vi "RF机柜开关切换.vi"(6 "COM":u16, 7 "A":u16, 8 "error in":errorcluster caption="error constant", 9 "8x4":refnum<k5>, 10 "RF-B":refnum<k5>, 11 "RF-A":refnum<k5>) -> (0 "error out":errorcluster caption="error constant", 2 "ask":string)   [LabVIEW 2015]
uses:
  server/Global/SeverGlobal.vi
panel:
  out "Isfailed":bool
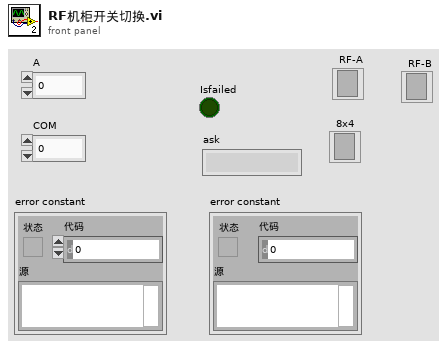
[diagram p1: front panel]
types:
  T1 = enum16{"Standard", "Buffered", "CRLF", "Immediate"}
  T2 = cluster{"IP_A":string, "PORT_A":i32, "IP_B":string, "PORT_B":i32, "IP_CLK":string, "PORT_CLK":i32, "IP_SWITCH":string, "PORT_SWITCH":i32}
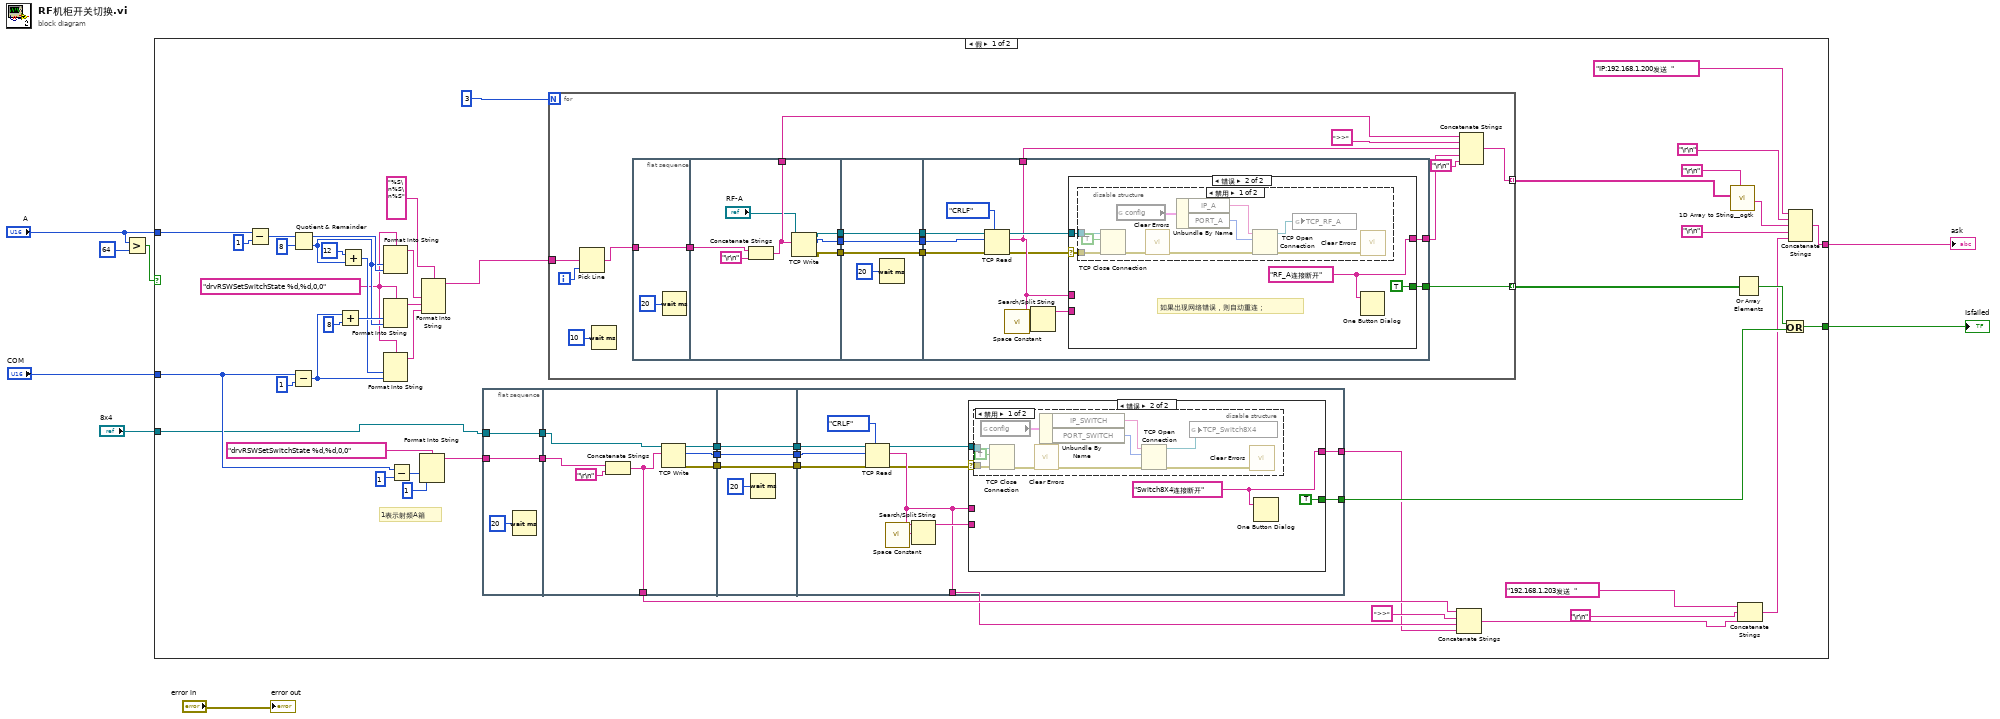
[diagram p0: block diagram]
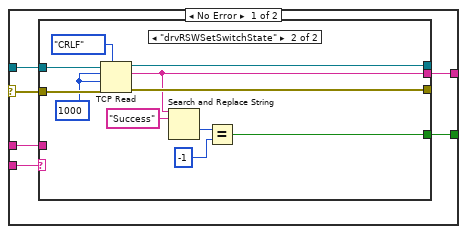
[diagram p2: hidden frame]
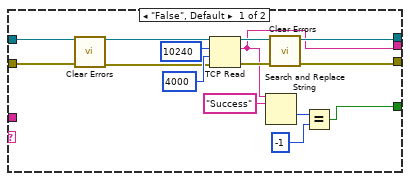
[diagram p3: hidden frame]
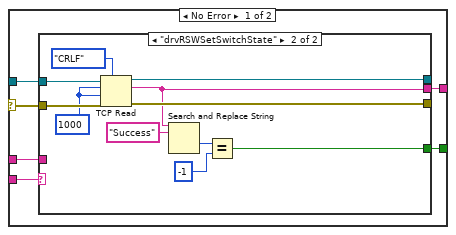
[diagram p5: hidden frame]
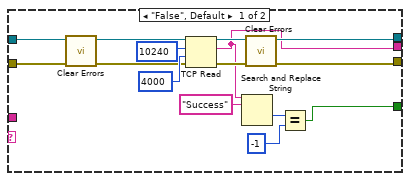
[diagram p6: hidden frame]
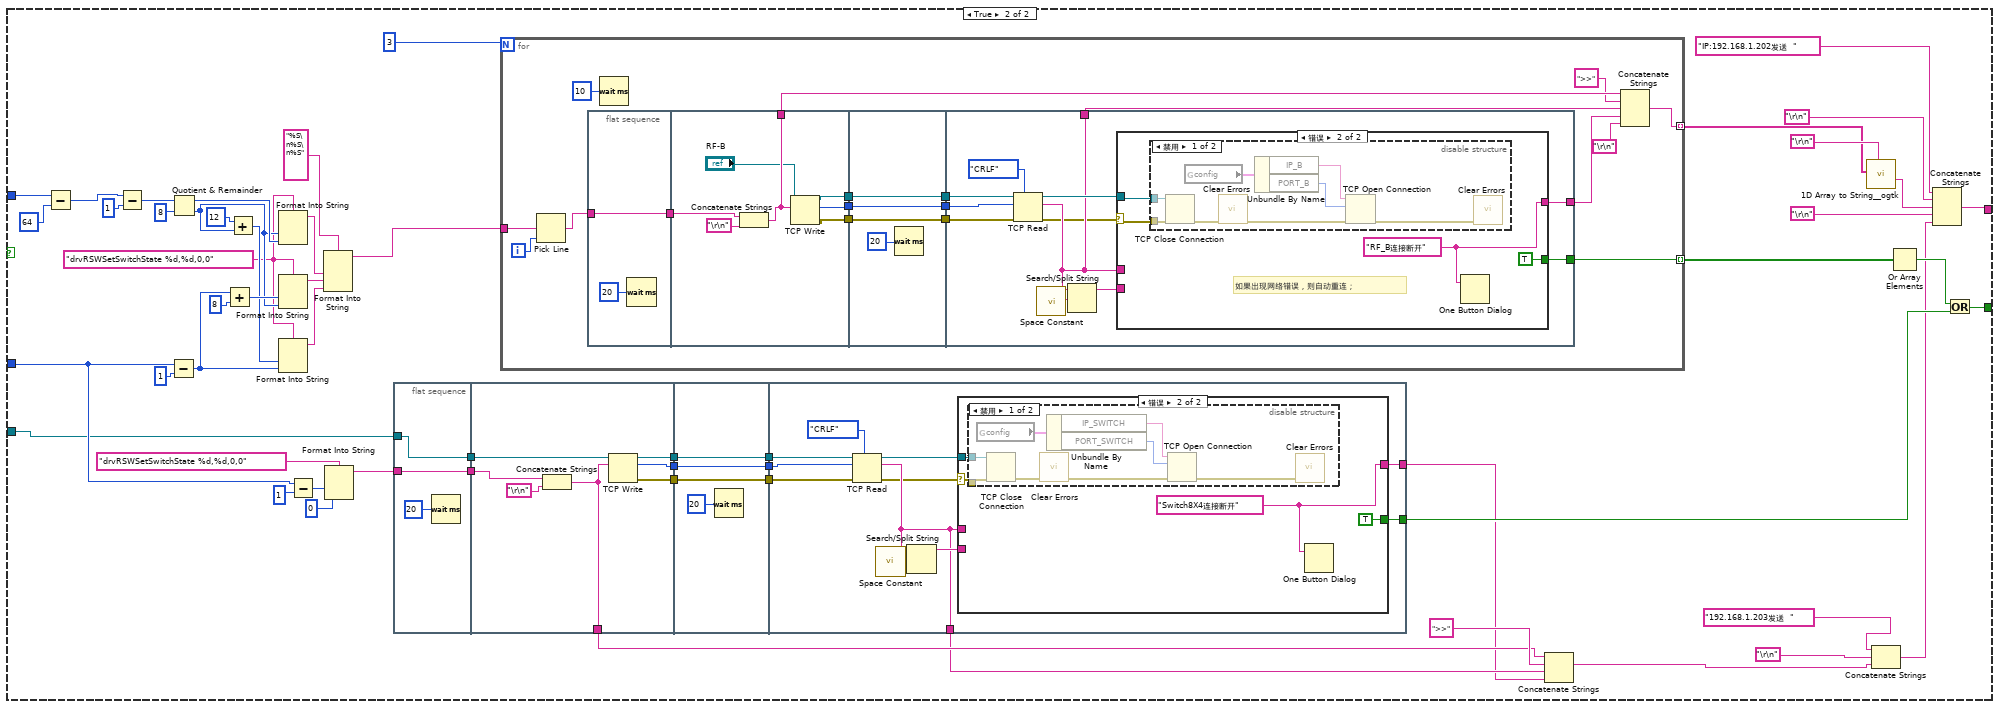
[diagram p8: hidden frame]
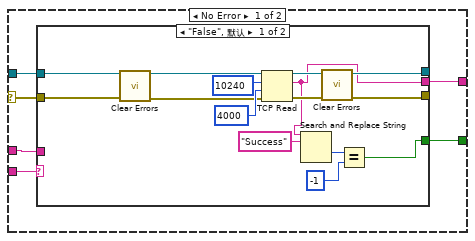
[diagram p9: hidden frame]
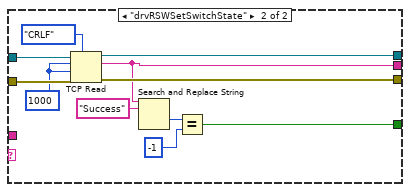
[diagram p10: hidden frame]
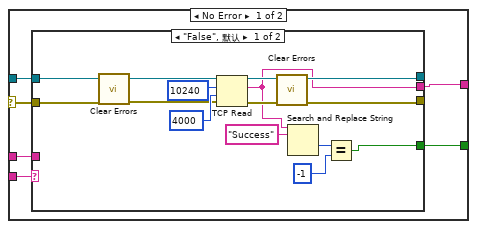
[diagram p12: hidden frame]
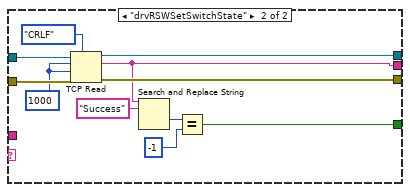
[diagram p13: hidden frame]
diagram:
  n1 = Greater?(x="A", y=u16 64) -> (0:w2:bool)
  n2 = case shown="假" w2 {
    tunnel: "A" -> [w43 w253]
    tunnel: "COM" -> [w39 w239]
    tunnel: [w27 w236] -> w5
    tunnel: [w24 w225] -> w4
    tunnel: "8x4" -> [w10 w218]
    frame False {
      w46 = "drvRSWSetSwitchState %d,%d,0,0" ("格式字符串")
      # "1表示射频A箱"
      n3 = Subtract(x=w43, y=1) -> (x-y=w60:i32)
      n4 = Subtract(x=w39, y=1) -> (x-y=w51:i32)
      n5 = Quotient & Remainder(x=w60, y=8) -> (x-y*floor(x/y)=w55:i32, floor(x/y)=w53:i32)
      n6 = Add(x=w51, y=8) -> (x+y=w54:i32)
      n7 = Add(x=12, y=w53) -> (x+y=w52:i32)
      n8 = Format Into String(format string=w46, w53, w55) -> (resulting string=w49:string)  [unwired: 2 in, 1 out]
      n9 = Format Into String(format string=w46, w54, w53) -> (resulting string=w48:string)  [unwired: 2 in, 1 out]
      n10 = Format Into String(format string=w46, w52, w51) -> (resulting string=w47:string)  [unwired: 2 in, 1 out]
      n11 = Subtract(x=w39, y=1) -> (x-y=w42:i32)
      n12 = Format Into String(format string="drvRSWSetSwitchState %d,%d,0,0" ("格式字符串"), w42, i16 1 ("input 2")) -> (resulting string=w37:string)  [unwired: 2 in, 1 out]
      n13 = Format Into String(format string="%S\n%S\n%S", w49, w48, w47) -> (resulting string=w45:string)  [unwired: 2 in, 1 out]
      n14 = flat-sequence {
        tunnel: w37 -> [w64]
        tunnel: [w64] -> w21
        tunnel: w10 -> [w62]
        tunnel: [w62] -> w9
        tunnel: [w69] -> w36
        tunnel: [w68] -> w35
        tunnel: [w67] -> w31
        tunnel: [w66] -> w14
        tunnel: w21 -> [w71]
        tunnel: w9 -> [w65]
        tunnel: w36 -> [w74]
        tunnel: w35 -> [w73]
        tunnel: [w74] -> w34
        tunnel: [w73] -> w33
        tunnel: [w72] -> w32
        tunnel: w31 -> [w72]
        tunnel: w34 -> [w82]
        tunnel: w33 -> [w81]
        tunnel: w32 -> [w80]
        tunnel: [w79] -> w28
        tunnel: [w78] -> w12
        tunnel: [w77] -> w13
        frame #0 {
          n15 = Wait (ms)(milliseconds to wait=u32 20 ("delay")) -> ()  [unwired: 1 out]
        }
        frame #1 {
          n16 = Concatenate Strings(w71, "\r\n") -> (w66:string)
          n17 = TCP Write(connection ID=w65, data in=w66) -> (connection ID out=w69:refnum<k5>, bytes written=w67:i32, error out=w68:errorcluster)  [unwired: 2 in]
        }
        frame #2 {
          n18 = Wait (ms)(milliseconds to wait=u32 20 ("delay")) -> ()  [unwired: 1 out]
        }
        frame #3 {
          n19 = TCP Read(connection ID=w82, bytes to read=w80, error in (no error)=w81, 7:T1."CRLF" ("mode (standard)")) -> (connection ID out=w86:refnum<k5>, data out=w77:string, error out=w76:errorcluster)  [unwired: 1 in]
          n20 = call <vilib>:"Space Constant.vi"() -> ("String"=w83:string)
          n21 = Search/Split String(string=w77, search string/char (-)=w83) -> (substring before match=w85:string)  [unwired: 1 in, 2 out]
          n22 = case shown="错误" w76 {
            selector: w76 -> [w87 w120]
            tunnel: w86 -> [w92 w119]
            tunnel: w85 -> [w91 _]
            tunnel: [w90 TRUE] -> w79
            tunnel: [w89 w117] -> w78
            tunnel: w77 -> [w88 _]
            frame No Error {
              n23 = case shown="\"drvRSWSetSwitchState\"" w91 {
                tunnel: [w101 w115] -> _
                tunnel: [w100 w114] -> _
                tunnel: w92 -> [w102 w113]
                tunnel: w87 -> [w99 w112]
                tunnel: w88 -> [_ _]
                tunnel: [w93 w107] -> w90
                tunnel: [w94 w106] -> w89
                frame "False", Default {
                  n24 = call <vilib>:"Clear Errors.vi"("error in (no error)"=w99) -> ("error out"=w98:errorcluster)  [unwired: 5 in, 1 out]
                  n25 = TCP Read(connection ID=w102, bytes to read=10240, error in (no error)=w98, 9:4000 ("timeout ms (25000)")) -> (connection ID out=w101:refnum<k5>, data out=w94:string, error out=w104:errorcluster)  [unwired: 1 in]
                  n26 = Search and Replace String(input string=w94, search string="Success") -> (offset past replacement=w95:i32)  [unwired: 6 in, 3 out]
                  n27 = call <vilib>:"Clear Errors.vi"("error in (no error)"=w104) -> ("error out"=w100:errorcluster)  [unwired: 5 in, 1 out]
                  n28 = Equal?(x=w95, y=-1) -> (x = y?=w93:bool)
                }
                frame "drvRSWSetSwitchState" {
                  w111 = 1000 ("timeout ms (25000)")
                  n29 = TCP Read(connection ID=w113, bytes to read=w111, error in (no error)=w112, 7:T1."CRLF" ("mode (standard)"), 9:w111) -> (connection ID out=w115:refnum<k5>, data out=w106:string, error out=w114:errorcluster)
                  n30 = Search and Replace String(input string=w106, search string="Success") -> (offset past replacement=w109:i32)  [unwired: 6 in, 3 out]
                  n31 = Equal?(x=w109, y=-1) -> (x = y?=w107:bool)
                }
              }
            }
            frame Error {
              w117 = "Switch8X4连接断开" ("字符串")
              n32 = disable-structure shown="禁用" {
                disable-tunnel: w120 -> [w123 _]
                disable-tunnel: w119 -> [w122 _]
                frame Disabled {
                  n33 = global read "SeverGlobal.vi" "config"() -> (w126:T2)
                  n34 = TCP Close Connection(connection ID=w122, abort (F)=TRUE ("中止(F)"), error in (no error)=w123) -> (error out=w124:errorcluster)  [unwired: 1 out]
                  n35 = call <vilib>:"Clear Errors.vi"("error in (no error)"=w124) -> ("error out"=w125:errorcluster)  [unwired: 5 in, 1 out]
                  n36 = Unbundle By Name(w126) -> ("IP_SWITCH"=w127:string, "PORT_SWITCH"=w128:i32)
                  n37 = TCP Open Connection(address=w127, remote port or service name=w128, error in (no error)=w125) -> (connection ID=w129:refnum<k5>, error out=w130:errorcluster)  [unwired: 2 in]
                  n38 = global write "SeverGlobal.vi" "TCP_Switch8X4"(w129) -> ()
                  n39 = call <vilib>:"Clear Errors.vi"("error in (no error)"=w130) -> ()  [unwired: 5 in, 2 out]
                }
                frame Enabled {
                }
              }
              n40 = One Button Dialog(message=w117) -> ()  [unwired: 1 in, 1 out]
            }
          }
        }
      }
      n41 = for {
        N: 3 -> [_]
        tunnel: w45 -> [w148]
        tunnel: [w138] -> w30 mode=indexing
        tunnel: [w135] -> w25 mode=indexing
        i -> [w147]
        n42 = Pick Line(multi-line string=w148, line index=w147) -> (output string=w146:string)  [unwired: 1 in]
        n43 = Wait (ms)(milliseconds to wait=u32 10 ("delay")) -> ()  [unwired: 1 out]
        n44 = flat-sequence {
          tunnel: w146 -> [w150]
          tunnel: [w150] -> w134
          tunnel: [w155] -> w144
          tunnel: [w154] -> w142
          tunnel: [w153] -> w140
          tunnel: [w152] -> w132
          tunnel: w134 -> [w156]
          tunnel: [w160] -> w145
          tunnel: w144 -> [w160]
          tunnel: [w159] -> w143
          tunnel: w142 -> [w159]
          tunnel: [w158] -> w141
          tunnel: w140 -> [w158]
          tunnel: w145 -> [w170]
          tunnel: w143 -> [w169]
          tunnel: w141 -> [w168]
          tunnel: [w165] -> w138
          tunnel: [w164] -> w137
          tunnel: [w163] -> w136
          frame #0 {
            n45 = Wait (ms)(milliseconds to wait=u32 20 ("delay")) -> ()  [unwired: 1 out]
          }
          frame #1 {
            n46 = Concatenate Strings(w156, "\r\n") -> (w152:string)
            n47 = TCP Write(connection ID="RF-A", data in=w152) -> (connection ID out=w155:refnum<k5>, bytes written=w154:i32, error out=w153:errorcluster)  [unwired: 2 in]
          }
          frame #2 {
            n48 = Wait (ms)(milliseconds to wait=u32 20 ("delay")) -> ()  [unwired: 1 out]
          }
          frame #3 {
            n49 = TCP Read(connection ID=w170, bytes to read=w169, error in (no error)=w168, 7:T1."CRLF" ("mode (standard)")) -> (connection ID out=w166:refnum<k5>, data out=w164:string, error out=w162:errorcluster)  [unwired: 1 in]
            n50 = call <vilib>:"Space Constant.vi"() -> ("String"=w172:string)
            n51 = Search/Split String(string=w164, search string/char (-)=w172) -> (substring before match=w167:string)  [unwired: 1 in, 2 out]
            n52 = case shown="错误" w162 {
              selector: w162 -> [w173 w205]
              tunnel: w167 -> [w178 _]
              tunnel: w166 -> [w177 w206]
              tunnel: [w176 TRUE] -> w165
              tunnel: w164 -> [w175 _]
              tunnel: [w174 w203] -> w163
              frame No Error {
                n53 = case shown="\"drvRSWSetSwitchState\"" w178 {
                  tunnel: [w187 w201] -> _
                  tunnel: [w186 w200] -> _
                  tunnel: w177 -> [w188 w199]
                  tunnel: w173 -> [w185 w198]
                  tunnel: w175 -> [_ _]
                  tunnel: [w179 w193] -> w176
                  tunnel: [w180 w192] -> w174
                  frame "False", Default {
                    n54 = call <vilib>:"Clear Errors.vi"("error in (no error)"=w185) -> ("error out"=w184:errorcluster)  [unwired: 5 in, 1 out]
                    n55 = TCP Read(connection ID=w188, bytes to read=10240, error in (no error)=w184, 9:4000 ("timeout ms (25000)")) -> (connection ID out=w187:refnum<k5>, data out=w180:string, error out=w190:errorcluster)  [unwired: 1 in]
                    n56 = Search and Replace String(input string=w180, search string="Success") -> (offset past replacement=w183:i32)  [unwired: 6 in, 3 out]
                    n57 = call <vilib>:"Clear Errors.vi"("error in (no error)"=w190) -> ("error out"=w186:errorcluster)  [unwired: 5 in, 1 out]
                    n58 = Equal?(x=w183, y=-1) -> (x = y?=w179:bool)
                  }
                  frame "drvRSWSetSwitchState" {
                    w197 = 1000 ("timeout ms (25000)")
                    n59 = TCP Read(connection ID=w199, bytes to read=w197, error in (no error)=w198, 7:T1."CRLF" ("mode (standard)"), 9:w197) -> (connection ID out=w201:refnum<k5>, data out=w192:string, error out=w200:errorcluster)
                    n60 = Search and Replace String(input string=w192, search string="Success") -> (offset past replacement=w195:i32)  [unwired: 6 in, 3 out]
                    n61 = Equal?(x=w195, y=-1) -> (x = y?=w193:bool)
                  }
                }
              }
              frame Error {
                w203 = "RF_A连接断开" ("字符串")
                # "如果出现网络错误，则自动重连；"
                n62 = disable-structure shown="禁用" {
                  disable-tunnel: w206 -> [w216 _]
                  disable-tunnel: w205 -> [w215 _]
                  frame Disabled {
                    n63 = TCP Close Connection(connection ID=w216, abort (F)=TRUE ("中止(F)"), error in (no error)=w215) -> (error out=w214:errorcluster)  [unwired: 1 out]
                    n64 = global read "SeverGlobal.vi" "config"() -> (w212:T2)
                    n65 = call <vilib>:"Clear Errors.vi"("error in (no error)"=w214) -> ("error out"=w213:errorcluster)  [unwired: 5 in, 1 out]
                    n66 = Unbundle By Name(w212) -> ("IP_A"=w211:string, "PORT_A"=w210:i32)
                    n67 = TCP Open Connection(address=w211, remote port or service name=w210, error in (no error)=w213) -> (connection ID=w209:refnum<k5>, error out=w208:errorcluster)  [unwired: 2 in]
                    n68 = global write "SeverGlobal.vi" "TCP_RF_A"(w209) -> ()
                    n69 = call <vilib>:"Clear Errors.vi"("error in (no error)"=w208) -> ()  [unwired: 5 in, 2 out]
                  }
                  frame Enabled {
                  }
                }
                n70 = One Button Dialog(message=w203) -> ()  [unwired: 1 in, 1 out]
              }
            }
          }
        }
        n71 = Concatenate Strings(w132, ">>" ("字符串"), w137, w136, "\r\n") -> (w135:string)
      }
      n72 = Concatenate Strings(w14, ">>" ("字符串"), w13, w12) -> (w11:string)
      n73 = call <userlib>:"1D Array to String__ogtk.vi"("delimiter (Tab)"="\r\n", "Array of Strings"=w25) -> ("delimited string"=w26:string)  [unwired: 9 in]
      n74 = Or Array Elements(Boolean array=w30) -> (logical OR=w29:bool)
      n75 = Concatenate Strings("192.168.1.203发送  " ("delimiter (Tab)"), "\r\n", w11) -> (w22:string)
      n76 = Or(x=w29, y=w28) -> (x .or. y?=w27:bool)
      n77 = Concatenate Strings("IP:192.168.1.200发送  " ("delimiter (Tab)"), "\r\n", w26, "\r\n", w22) -> (w24:string)
    }
    frame True {
      w256 = "drvRSWSetSwitchState %d,%d,0,0" ("格式字符串")
      n78 = Subtract(x=w253, y=u16 64) -> (x-y=w251:u16)
      n79 = Subtract(x=w251, y=1) -> (x-y=w270:i32)
      n80 = Subtract(x=w239, y=1) -> (x-y=w261:i32)
      n81 = Quotient & Remainder(x=w270, y=8) -> (x-y*floor(x/y)=w265:i32, floor(x/y)=w263:i32)
      n82 = Add(x=w261, y=8) -> (x+y=w264:i32)
      n83 = Add(x=12, y=w263) -> (x+y=w262:i32)
      n84 = Format Into String(format string=w256, w263, w265) -> (resulting string=w259:string)  [unwired: 2 in, 1 out]
      n85 = Format Into String(format string=w256, w264, w263) -> (resulting string=w258:string)  [unwired: 2 in, 1 out]
      n86 = Format Into String(format string=w256, w262, w261) -> (resulting string=w257:string)  [unwired: 2 in, 1 out]
      n87 = Subtract(x=w239, y=1) -> (x-y=w244:i32)
      n88 = Format Into String(format string="%S\n%S\n%S", w259, w258, w257) -> (resulting string=w255:string)  [unwired: 2 in, 1 out]
      n89 = Format Into String(format string="drvRSWSetSwitchState %d,%d,0,0" ("格式字符串"), w244, i16 0 ("input 2")) -> (resulting string=w240:string)  [unwired: 2 in, 1 out]
      n90 = flat-sequence {
        tunnel: w240 -> [w274]
        tunnel: [w274] -> w233
        tunnel: w218 -> [w272]
        tunnel: [w272] -> w217
        tunnel: [w279] -> w250
        tunnel: [w278] -> w249
        tunnel: [w277] -> w248
        tunnel: [w276] -> w223
        tunnel: w233 -> [w281]
        tunnel: w217 -> [w275]
        tunnel: w250 -> [w284]
        tunnel: w249 -> [w283]
        tunnel: [w284] -> w247
        tunnel: [w283] -> w246
        tunnel: [w282] -> w245
        tunnel: w248 -> [w282]
        tunnel: w247 -> [w292]
        tunnel: w246 -> [w291]
        tunnel: w245 -> [w290]
        tunnel: [w289] -> w235
        tunnel: [w288] -> w222
        tunnel: [w287] -> w221
        frame #0 {
          n91 = Wait (ms)(milliseconds to wait=u32 20 ("delay")) -> ()  [unwired: 1 out]
        }
        frame #1 {
          n92 = Concatenate Strings(w281, "\r\n") -> (w276:string)
          n93 = TCP Write(connection ID=w275, data in=w276) -> (connection ID out=w279:refnum<k5>, bytes written=w277:i32, error out=w278:errorcluster)  [unwired: 2 in]
        }
        frame #2 {
          n94 = Wait (ms)(milliseconds to wait=u32 20 ("delay")) -> ()  [unwired: 1 out]
        }
        frame #3 {
          n95 = TCP Read(connection ID=w292, bytes to read=w290, error in (no error)=w291, 7:T1."CRLF" ("mode (standard)")) -> (connection ID out=w296:refnum<k5>, data out=w288:string, error out=w286:errorcluster)  [unwired: 1 in]
          n96 = call <vilib>:"Space Constant.vi"() -> ("String"=w293:string)
          n97 = Search/Split String(string=w288, search string/char (-)=w293) -> (substring before match=w295:string)  [unwired: 1 in, 2 out]
          n98 = case shown="错误" w286 {
            selector: w286 -> [w297 w330]
            tunnel: w296 -> [w302 w329]
            tunnel: w295 -> [w301 _]
            tunnel: [w300 TRUE] -> w289
            tunnel: w288 -> [w299 _]
            tunnel: [w298 w327] -> w287
            frame No Error {
              n99 = case shown="\"False\", 默认" w301 {
                tunnel: [w311 w325] -> _
                tunnel: [w310 w324] -> _
                tunnel: w302 -> [w312 w323]
                tunnel: w297 -> [w309 w322]
                tunnel: w299 -> [_ _]
                tunnel: [w303 w317] -> w300
                tunnel: [w305 w316] -> w298
                frame "False", Default {
                  n100 = call <vilib>:"Clear Errors.vi"("error in (no error)"=w309) -> ("error out"=w308:errorcluster)  [unwired: 5 in, 1 out]
                  n101 = TCP Read(connection ID=w312, bytes to read=10240, error in (no error)=w308, 9:4000 ("timeout ms (25000)")) -> (connection ID out=w311:refnum<k5>, data out=w305:string, error out=w314:errorcluster)  [unwired: 1 in]
                  n102 = Search and Replace String(input string=w305, search string="Success") -> (offset past replacement=w306:i32)  [unwired: 6 in, 3 out]
                  n103 = call <vilib>:"Clear Errors.vi"("error in (no error)"=w314) -> ("error out"=w310:errorcluster)  [unwired: 5 in, 1 out]
                  n104 = Equal?(x=w306, y=-1) -> (x = y?=w303:bool)
                }
                frame "drvRSWSetSwitchState" {
                  w321 = 1000 ("timeout ms (25000)")
                  n105 = TCP Read(connection ID=w323, bytes to read=w321, error in (no error)=w322, 7:T1."CRLF" ("mode (standard)"), 9:w321) -> (connection ID out=w325:refnum<k5>, data out=w316:string, error out=w324:errorcluster)
                  n106 = Search and Replace String(input string=w316, search string="Success") -> (offset past replacement=w319:i32)  [unwired: 6 in, 3 out]
                  n107 = Equal?(x=w319, y=-1) -> (x = y?=w317:bool)
                }
              }
            }
            frame Error {
              w327 = "Switch8X4连接断开" ("字符串")
              n108 = disable-structure shown="禁用" {
                disable-tunnel: w330 -> [w332 _]
                disable-tunnel: w329 -> [w331 _]
                frame Disabled {
                  n109 = global read "SeverGlobal.vi" "config"() -> (w335:T2)
                  n110 = TCP Close Connection(connection ID=w331, error in (no error)=w332) -> (error out=w333:errorcluster)  [unwired: 1 in, 1 out]
                  n111 = call <vilib>:"Clear Errors.vi"("error in (no error)"=w333) -> ("error out"=w334:errorcluster)  [unwired: 5 in, 1 out]
                  n112 = Unbundle By Name(w335) -> ("IP_SWITCH"=w336:string, "PORT_SWITCH"=w337:i32)
                  n113 = TCP Open Connection(address=w336, remote port or service name=w337, error in (no error)=w334) -> (error out=w338:errorcluster)  [unwired: 2 in, 1 out]
                  n114 = call <vilib>:"Clear Errors.vi"("error in (no error)"=w338) -> ()  [unwired: 5 in, 2 out]
                }
                frame Enabled {
                }
              }
              n115 = One Button Dialog(message=w327) -> ()  [unwired: 1 in, 1 out]
            }
          }
        }
      }
      n116 = for {
        N: 3 -> [_]
        tunnel: w255 -> [w356]
        tunnel: [w347] -> w237 mode=indexing
        tunnel: [w339] -> w227 mode=indexing
        i -> [w355]
        n117 = Pick Line(multi-line string=w356, line index=w355) -> (output string=w354:string)  [unwired: 1 in]
        n118 = flat-sequence {
          tunnel: w354 -> [w358]
          tunnel: [w358] -> w346
          tunnel: [w363] -> w352
          tunnel: [w362] -> w350
          tunnel: [w361] -> w348
          tunnel: [w360] -> w343
          tunnel: w346 -> [w364]
          tunnel: [w368] -> w353
          tunnel: w352 -> [w368]
          tunnel: [w367] -> w351
          tunnel: w350 -> [w367]
          tunnel: [w366] -> w349
          tunnel: w348 -> [w366]
          tunnel: w353 -> [w378]
          tunnel: w351 -> [w377]
          tunnel: w349 -> [w376]
          tunnel: [w373] -> w347
          tunnel: [w372] -> w341
          tunnel: [w371] -> w340
          frame #0 {
            n119 = Wait (ms)(milliseconds to wait=u32 20 ("delay")) -> ()  [unwired: 1 out]
          }
          frame #1 {
            n120 = Concatenate Strings(w364, "\r\n") -> (w360:string)
            n121 = TCP Write(connection ID="RF-B", data in=w360) -> (connection ID out=w363:refnum<k5>, bytes written=w362:i32, error out=w361:errorcluster)  [unwired: 2 in]
          }
          frame #2 {
            n122 = Wait (ms)(milliseconds to wait=u32 20 ("delay")) -> ()  [unwired: 1 out]
          }
          frame #3 {
            n123 = TCP Read(connection ID=w378, bytes to read=w377, error in (no error)=w376, 7:T1."CRLF" ("mode (standard)")) -> (connection ID out=w374:refnum<k5>, data out=w372:string, error out=w370:errorcluster)  [unwired: 1 in]
            n124 = call <vilib>:"Space Constant.vi"() -> ("String"=w380:string)
            n125 = Search/Split String(string=w372, search string/char (-)=w380) -> (substring before match=w375:string)  [unwired: 1 in, 2 out]
            n126 = case shown="错误" w370 {
              selector: w370 -> [w381 w414]
              tunnel: w375 -> [w386 _]
              tunnel: w374 -> [w385 w413]
              tunnel: [w384 TRUE] -> w373
              tunnel: w372 -> [w383 _]
              tunnel: [w382 w411] -> w371
              frame No Error {
                n127 = case shown="\"False\", 默认" w386 {
                  tunnel: [w395 w409] -> _
                  tunnel: [w394 w408] -> _
                  tunnel: w385 -> [w396 w407]
                  tunnel: w381 -> [w393 w406]
                  tunnel: w383 -> [_ _]
                  tunnel: [w387 w401] -> w384
                  tunnel: [w388 w400] -> w382
                  frame "False", Default {
                    n128 = call <vilib>:"Clear Errors.vi"("error in (no error)"=w393) -> ("error out"=w392:errorcluster)  [unwired: 5 in, 1 out]
                    n129 = TCP Read(connection ID=w396, bytes to read=10240, error in (no error)=w392, 9:4000 ("timeout ms (25000)")) -> (connection ID out=w395:refnum<k5>, data out=w388:string, error out=w398:errorcluster)  [unwired: 1 in]
                    n130 = call <vilib>:"Clear Errors.vi"("error in (no error)"=w398) -> ("error out"=w394:errorcluster)  [unwired: 5 in, 1 out]
                    n131 = Search and Replace String(input string=w388, search string="Success") -> (offset past replacement=w390:i32)  [unwired: 6 in, 3 out]
                    n132 = Equal?(x=w390, y=-1) -> (x = y?=w387:bool)
                  }
                  frame "drvRSWSetSwitchState" {
                    w405 = 1000 ("timeout ms (25000)")
                    n133 = TCP Read(connection ID=w407, bytes to read=w405, error in (no error)=w406, 7:T1."CRLF" ("mode (standard)"), 9:w405) -> (connection ID out=w409:refnum<k5>, data out=w400:string, error out=w408:errorcluster)
                    n134 = Search and Replace String(input string=w400, search string="Success") -> (offset past replacement=w403:i32)  [unwired: 6 in, 3 out]
                    n135 = Equal?(x=w403, y=-1) -> (x = y?=w401:bool)
                  }
                }
              }
              frame Error {
                w411 = "RF_B连接断开" ("字符串")
                # "如果出现网络错误，则自动重连；"
                n136 = disable-structure shown="禁用" {
                  disable-tunnel: w414 -> [w416 _]
                  disable-tunnel: w413 -> [w415 _]
                  frame Disabled {
                    n137 = TCP Close Connection(connection ID=w415, error in (no error)=w416) -> (error out=w417:errorcluster)  [unwired: 1 in, 1 out]
                    n138 = global read "SeverGlobal.vi" "config"() -> (w419:T2)
                    n139 = call <vilib>:"Clear Errors.vi"("error in (no error)"=w417) -> ("error out"=w418:errorcluster)  [unwired: 5 in, 1 out]
                    n140 = Unbundle By Name(w419) -> ("IP_B"=w420:string, "PORT_B"=w421:i32)
                    n141 = TCP Open Connection(address=w420, remote port or service name=w421, error in (no error)=w418) -> (error out=w422:errorcluster)  [unwired: 2 in, 1 out]
                    n142 = call <vilib>:"Clear Errors.vi"("error in (no error)"=w422) -> ()  [unwired: 5 in, 2 out]
                  }
                  frame Enabled {
                  }
                }
                n143 = One Button Dialog(message=w411) -> ()  [unwired: 1 in, 1 out]
              }
            }
          }
        }
        n144 = Wait (ms)(milliseconds to wait=u32 10 ("delay")) -> ()  [unwired: 1 out]
        n145 = Concatenate Strings(w343, ">>" ("字符串"), w341, w340, "\r\n") -> (w339:string)
      }
      n146 = Concatenate Strings(w223, ">>" ("字符串"), w222, w221) -> (w219:string)
      n147 = call <userlib>:"1D Array to String__ogtk.vi"("delimiter (Tab)"="\r\n", "Array of Strings"=w227) -> ("delimited string"=w232:string)  [unwired: 9 in]
      n148 = Concatenate Strings("192.168.1.203发送  " ("delimiter (Tab)"), "\r\n", w219) -> (w226:string)
      n149 = Or Array Elements(Boolean array=w237) -> (logical OR=w238:bool)
      n150 = Concatenate Strings("IP:192.168.1.202发送  " ("delimiter (Tab)"), "\r\n", w232, "\r\n", w226) -> (w225:string)
      n151 = Or(x=w238, y=w235) -> (x .or. y?=w236:bool)
    }
  }
  "Isfailed" <- w5
  "ask" <- w4
  "error out" <- "error in"
